vi "Example.vi"() -> ()   [LabVIEW 2009]
panel:
  out "Mapped Data Visual out":T1(graph)
  out "Robot pos new":dbl[](array[numeric])
  in  "select map file":path
  out "LRF out":dbl[](graph)
  in  "rotation rate (w) in":dbl(slide)=0.020202020202020034 scale=4.0..-4.0
  in  "velocity (v) in":dbl(slide)=2.0 scale=-200.0..8000.0
  in  "stop":bool
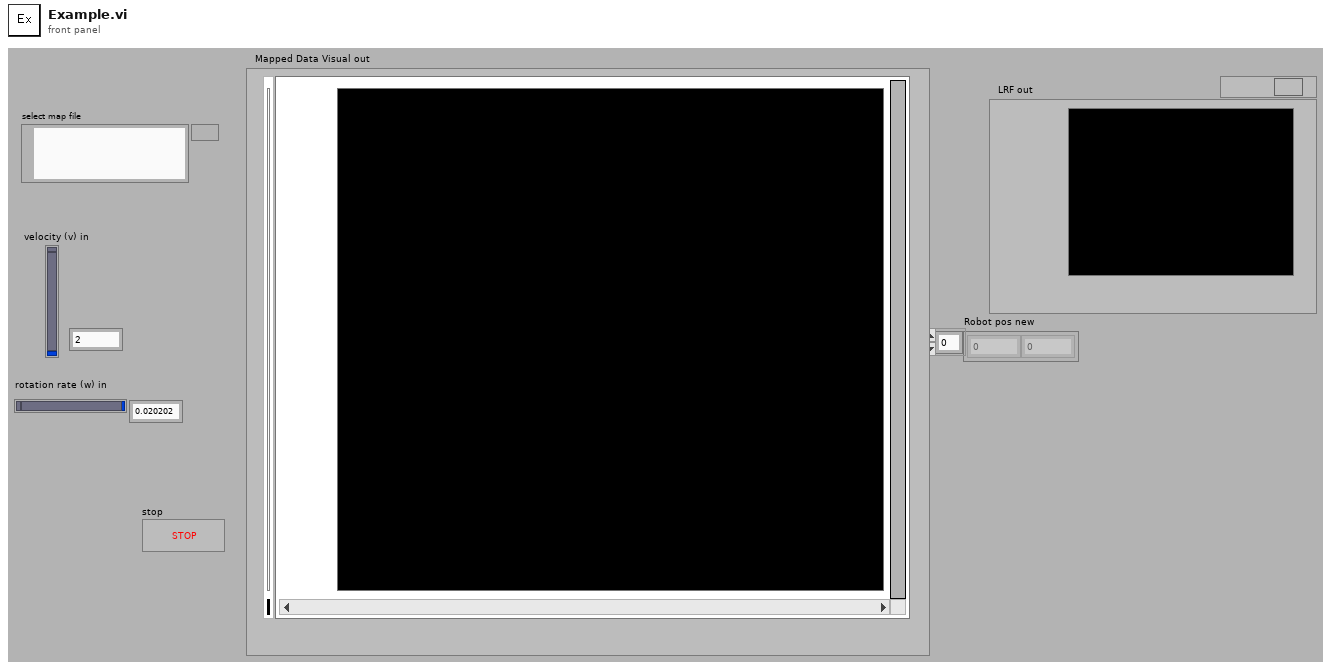
[diagram p1: front panel]
types:
  T1 = cluster{cluster{dbl[], dbl[]}, "output cluster":cluster{dbl[], dbl[]}, cluster{dbl[], dbl[]}, cluster{dbl[], dbl[]}, cluster{dbl[], dbl[]}, cluster{dbl[], dbl[]}, cluster{dbl[], dbl[]}}
  T2 = cluster{"P1x":dbl[], "P1y":dbl[], "P2x":dbl[], "P2y":dbl[], "Circ x":dbl[], "Circ y":dbl[], "Radius":dbl[], "LX":dbl[], "LY":dbl[], "CX":dbl[], "CY":dbl[], "Blue Flag x":dbl[], "Blue Flag y":dbl[], "Red Flag x":dbl[], "Red Flag y":dbl[], "GPS waypoint x":dbl[], "GPS waypoint y":dbl[]}
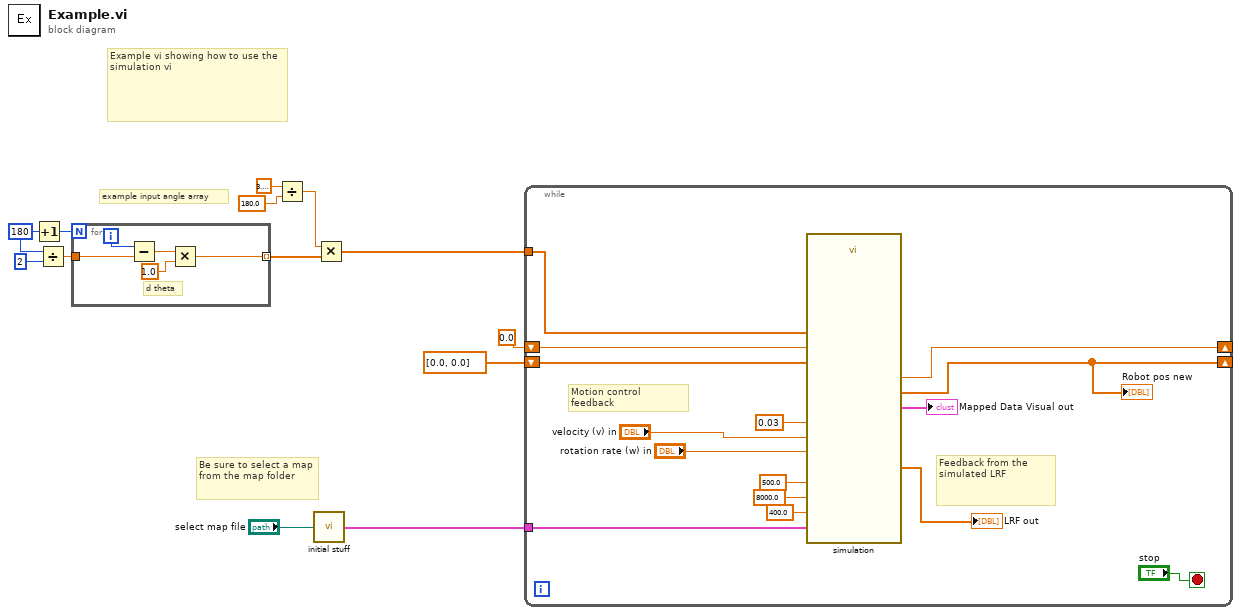
[diagram p0: block diagram]
diagram:
  w4 = 180
  # "Be sure to select a map from the map folder"
  # "Example vi showing how to use the simulation vi"
  # "example input angle array"
  n1 = Increment(x=w4) -> (x+1=w3:i32)
  n2 = Divide(x=w4, y=2) -> (x/y=w12:dbl)
  n3 = for {
    N: w3 -> [_]
    tunnel: w12 -> [w17]
    tunnel: [w14] -> w2 mode=indexing
    i -> [w18]
    # "d theta"
    n4 = Subtract(x=w18, y=w17) -> (x-y=w16:dbl)
    n5 = Multiply(x=w16, y=1.0) -> (x*y=w14:dbl)
  }
  n6 = Divide(x=3.141592653589793, y=180.0) -> (x/y=w9:dbl)
  n7 = call "initial stuff.vi"("select file"="select map file") -> ("Map Data"=w1:T2)
  n8 = Multiply(x=w9, y=w2) -> (x*y=w8:dbl[])
  n9 = while {
    tunnel: w8 -> [w33]
    shift-right: [w31] -> _
    shift-left: dbl[] [0.0, 0.0] ("R pos new") -> [w30]
    shift-right: [w29] -> _
    shift-left: 0.0 ("R dir new") -> [w28]
    tunnel: w1 -> [w20]
    stop <- "stop" stop-if-true
    # "Feedback from the simulated LRF"
    # "Motion control feedback"
    n10 = call "simulation.vi"("Angle"=w33, "dt"=0.03, "Map Data"=w20, "R dir"=w28, "Robot Radius"=500.0, "R pos"=w30, "LRF range"=8000.0 ("max dist"), "w"="rotation rate (w) in", "LRF offset"=400.0, "v"="velocity (v) in") -> ("Mapped Data Visual out"=→"Mapped Data Visual out":T1, "Robot pos new"=w31:dbl[], "Robot dir new"=w29:dbl, "LRF"=→"LRF out":dbl[])  [unwired: 2 in]
    "Robot pos new" <- w31
  }
